vi "Plot Maximize Button Exists.vi"(8 "error in (no error)":errorcluster, 11 "StokePlotHandle in":refnum<class "BjusticePlotHandle.lvclass">) -> (0 "error out":errorcluster, 2 "Plot Maximize Button exists?":bool, 3 "StokePlotHandle out":refnum<class "BjusticePlotHandle.lvclass">)   [LabVIEW 2021, in "BjusticePlotHandle.lvclass"]
uses:
  BjusticePlotHandle.lvclass
  BjusticePlotHandle.lvclass/BjusticePlotHandle.ctl
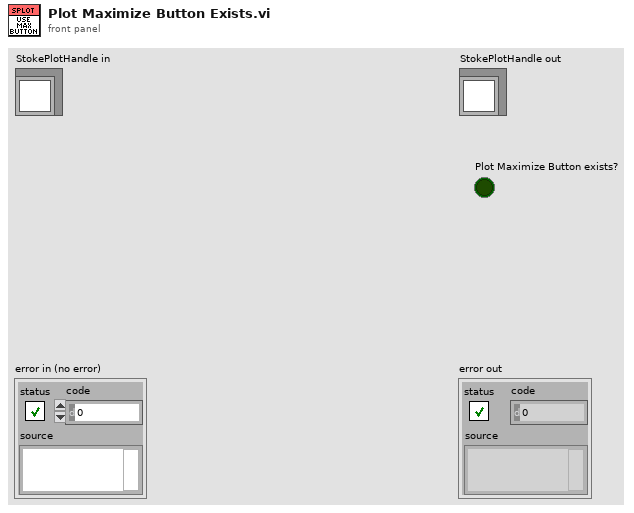
[diagram p1: front panel]
types:
  T1 = typedef "StokePlotHandle.lvclass/Type.ctl" = enum16{"1PLOT", "MPLOT"}
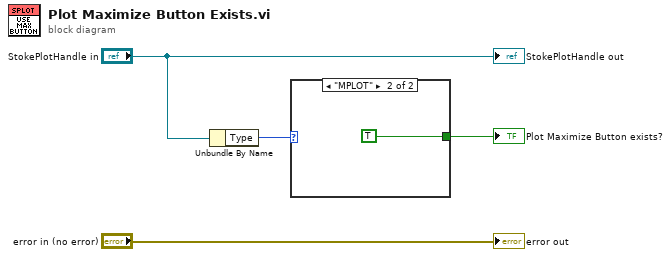
[diagram p0: block diagram]
diagram:
  n1 = Unbundle By Name("StokePlotHandle in") -> ("Type"=w2:T1)
  n2 = case shown="\"MPLOT\"" w2 {
    tunnel: [_ TRUE] -> w1
    frame "1PLOT" {
    }
    frame "MPLOT" {
    }
  }
  "Plot Maximize Button exists?" <- w1
  "error out" <- "error in (no error)"
  "StokePlotHandle out" <- "StokePlotHandle in"
